vi "Exclusion Data From Tree.vi"(8 "error in":errorcluster, 11 "XML in":string) -> (0 "error out":errorcluster, 2 "Exclusion Data":T1[](array[typedef]), 3 "XML out":string)   [LabVIEW 2020]
uses:
  <vilib>/addons/analyzer/_analyzerctrls.llb/VIAnCtl Exclusion Data.ctl
  <vilib>/addons/analyzer/_vianuishared.llb/VIAnUI CFG File Info Global.vi
  <vilib>/addons/analyzer/XML Parsing/NI_VIAn_XML Parsing.lvlib
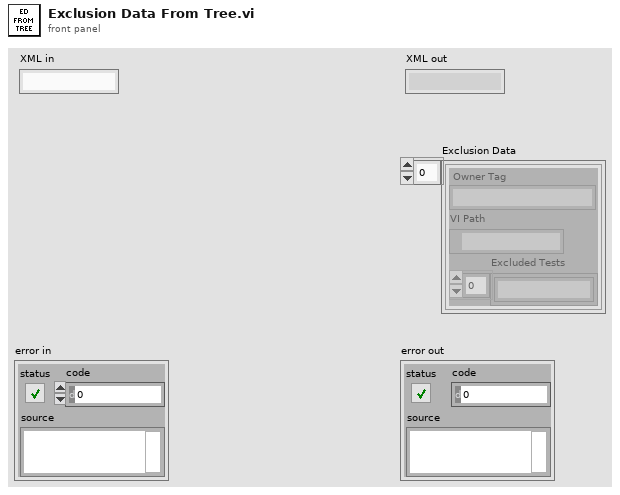
[diagram p1: front panel]
types:
  T1 = typedef "VIAnCtl Exclusion Data.ctl" = cluster{"Owner Tag":string, "VI Path":path, "Excluded Tests":string[]}
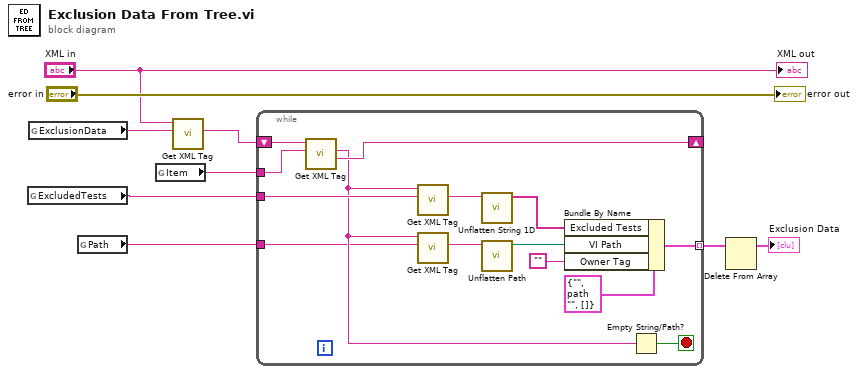
[diagram p0: block diagram]
diagram:
  n1 = global read "VIAnUI CFG File Info Global.vi" "ExcludedTests"() -> (w2:string)
  n2 = global read "VIAnUI CFG File Info Global.vi" "ExclusionData"() -> (w7:string)
  n3 = global read "VIAnUI CFG File Info Global.vi" "Path"() -> (w1:string)
  n4 = global read "VIAnUI CFG File Info Global.vi" "Item"() -> (w3:string)
  n5 = call <vilib>:"Get XML Tag.vi"("Tag name"=w7, "XML String in"="XML in") -> ("Tag value"=w6:string)  [unwired: 5 in, 4 out]
  n6 = while {
    tunnel: [w22] -> w5 mode=indexing
    shift-right: [w19] -> _
    shift-left: w6 -> [w20]
    tunnel: w3 -> [w18]
    tunnel: w2 -> [w16]
    tunnel: w1 -> [w14]
    stop <- w17 stop-if-true
    n7 = call <vilib>:"Get XML Tag.vi"("Tag name"=w18, "XML String in"=w20) -> ("Remaining string"=w19:string, "Tag value"=w15:string)  [unwired: 5 in, 3 out]
    n8 = call <vilib>:"Get XML Tag.vi"("Tag name"=w16, "XML String in"=w15) -> ("Tag value"=w11:string)  [unwired: 5 in, 4 out]
    n9 = call <vilib>:"Get XML Tag.vi"("Tag name"=w14, "XML String in"=w15) -> ("Tag value"=w13:string)  [unwired: 5 in, 4 out]
    n10 = call <vilib>:"Unflatten String 1D.vi"("Tag value"=w11) -> ("String Array 1D"=w10:string[])  [unwired: 10 in]
    n11 = call <vilib>:"Unflatten Path.vi"("Tag value"=w13) -> ("Path"=w12:path)  [unwired: 10 in]
    n12 = Bundle By Name(cluster=T1 {"Owner Tag"="", "VI Path"=path "", "Excluded Tests"=[]} ("Data"), "Excluded Tests"=w10, "VI Path"=w12, "Owner Tag"="") -> (w22:T1)
    n13 = Empty String/Path?(string/path=w15) -> (empty?=w17:bool)
  }
  n14 = Delete From Array(array=w5) -> (array with subset deleted=→"Exclusion Data":T1[])  [unwired: 2 in, 1 out]
  "error out" <- "error in"
  "XML out" <- "XML in"
